vi "ATF-Log command to DR.vi"(8 "error in (no error)":errorcluster, 11 "Cluster":T1) -> (0 "error out":errorcluster)   [LabVIEW 2022 SP3]
uses:
  Controls/SeCrTs-Notifier ctl.ctl
  Controls/SeCrTs-NS Data type.ctl
  Controls/Commands to Log monitor.ctl
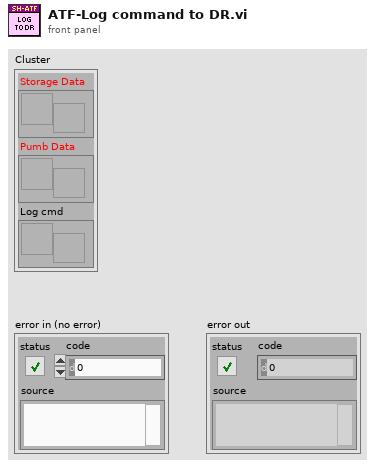
[diagram p1: front panel]
types:
  T1 = typedef "SeCrTs-Notifier ctl.ctl" = cluster{"Storage Data":refnum<notifier>, "Pumb Data":refnum<notifier>, "Log cmd":refnum<notifier>}
  T2 = cluster{"listener ID":refnum<k5>, "connection ID":refnum<k5>, "Log CMD":refnum<notifier>, "Data":cluster{"C/NC":bool, "Start/Stop Log":bool[], "Log Name":string, "Config":cluster{"AO config":cluster{"Channel_Name":string, "Channel_Number":string, "Default_Value":dbl, "Units":string}[], "AI config":cluster{"Channel_Name":string, "Channel_Number":string, "Pre_Scale_min":dbl, "Pre_Scale_max":dbl, "Sensor_min":dbl, "Sensor_max":dbl, "Units":string}[], "DI config":cluster{"Channel_Name":string, "Channel_Number":string, "Default_Value":bool, "DI invert?":bool}[], "DO config":cluster{"Channel_Name":string, "Channel_Number":string, "Default_Value":bool, "DO invert?":bool}[], "TC config":cluster{"Channel_Name":string, "Channel_Number":string, "Pre_Scale_min":dbl, "Pre_Scale_max":dbl, "units":i32, " type":i32}[], "ACC config":cluster{"Channel_Name":string, "Channel_Number":string, "Pre_Scale_min":dbl, "Pre_Scale_max":dbl, "Terminal configuration":i32, "Sensitivity":dbl, "Sensitivity units":i32}[], "SG config":cluster{"Channel_Name":string, "Channel_Number":string, "Pre_Scale_min":dbl, "Pre_Scale_max":dbl}[], "Strain Gauge Settings":cluster{"poisson ratio":dbl, "nominal gage resistance":dbl, "gage factor":dbl}, "Bridge Settings":cluster{"voltage excitation value":dbl, "voltage excitation source":i32, "initial bridge voltage":dbl, "lead wire resistance":dbl, "strain configuration":i32}, "Sample Rate":cluster{"AI Sample Rate":dbl[], "AO Sample Rate":dbl[], "DI Sample Rate":dbl[], "TC Sample Rate":dbl[], "DO Sample Rate":dbl[], "SG Sample Rate":dbl[], "ACC Sample Rate":dbl[]}}, "Log min":dbl}, "timeout":i32}
  T3 = typedef "Commands to Log monitor.ctl" = enum16{"initialize", "Close", "Wait on Listener", "Write", "exit"}
  T4 = cluster{"C/NC":bool, "Start/Stop Log":bool[], "Log Name":string, "Config":cluster{"AO config":cluster{"Channel_Name":string, "Channel_Number":string, "Default_Value":dbl, "Units":string}[], "AI config":cluster{"Channel_Name":string, "Channel_Number":string, "Pre_Scale_min":dbl, "Pre_Scale_max":dbl, "Sensor_min":dbl, "Sensor_max":dbl, "Units":string}[], "DI config":cluster{"Channel_Name":string, "Channel_Number":string, "Default_Value":bool, "DI invert?":bool}[], "DO config":cluster{"Channel_Name":string, "Channel_Number":string, "Default_Value":bool, "DO invert?":bool}[], "TC config":cluster{"Channel_Name":string, "Channel_Number":string, "Pre_Scale_min":dbl, "Pre_Scale_max":dbl, "units":i32, " type":i32}[], "ACC config":cluster{"Channel_Name":string, "Channel_Number":string, "Pre_Scale_min":dbl, "Pre_Scale_max":dbl, "Terminal configuration":i32, "Sensitivity":dbl, "Sensitivity units":i32}[], "SG config":cluster{"Channel_Name":string, "Channel_Number":string, "Pre_Scale_min":dbl, "Pre_Scale_max":dbl}[], "Strain Gauge Settings":cluster{"poisson ratio":dbl, "nominal gage resistance":dbl, "gage factor":dbl}, "Bridge Settings":cluster{"voltage excitation value":dbl, "voltage excitation source":i32, "initial bridge voltage":dbl, "lead wire resistance":dbl, "strain configuration":i32}, "Sample Rate":cluster{"AI Sample Rate":dbl[], "AO Sample Rate":dbl[], "DI Sample Rate":dbl[], "TC Sample Rate":dbl[], "DO Sample Rate":dbl[], "SG Sample Rate":dbl[], "ACC Sample Rate":dbl[]}}, "Log min":dbl}
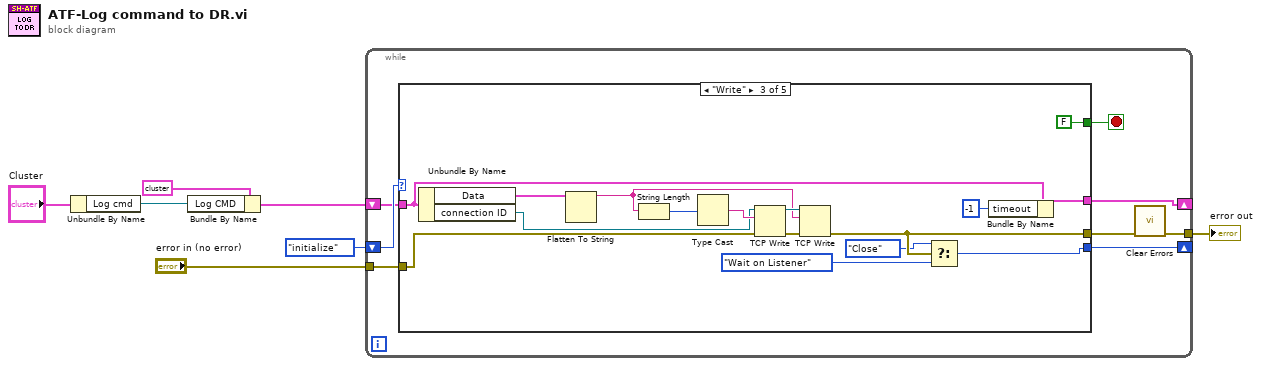
[diagram p0: block diagram]
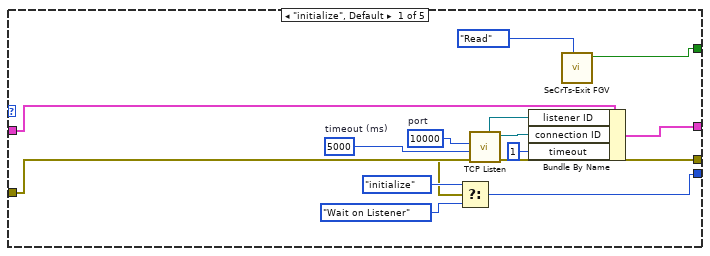
[diagram p2: hidden frame]
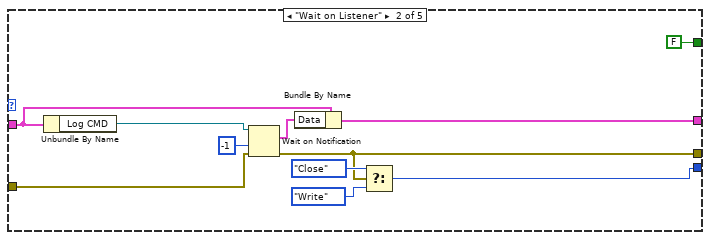
[diagram p3: hidden frame]
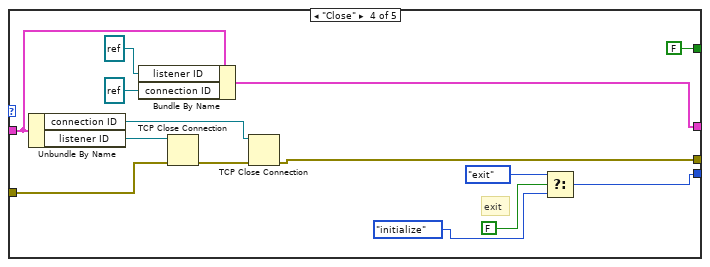
[diagram p4: hidden frame]
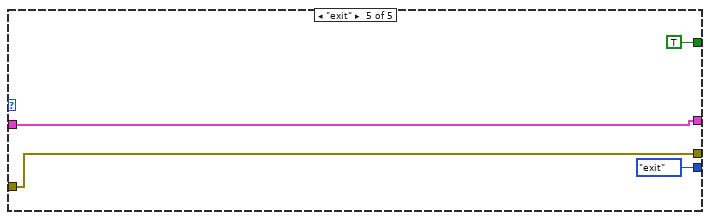
[diagram p5: hidden frame]
diagram:
  n1 = Unbundle By Name("Cluster") -> ("Log cmd"=w1:refnum<notifier>)
  n2 = Bundle By Name(cluster=T2 {"listener ID"=refnum, "connection ID"=refnum, "Log CMD"=refnum, "Data"={"C/NC"=FALSE, "Start/Stop Log"=[], "Log Name"="", "Config"={"AO config"=[], "AI config"=[], "DI config"=[], "DO config"=[], "TC config"=[], "ACC config"=[], "SG config"=[], "Strain Gauge Settings"={"poisson ratio"=0.0, "nominal gage resistance"=0.0, "gage factor"=0.0}, "Bridge Settings"={"voltage excitation value"=0.0, "voltage excitation source"=0, "initial bridge voltage"=0.0, "lead wire resistance"=0.0, "strain configuration"=0}, "Sample Rate"={"AI Sample Rate"=[], "AO Sample Rate"=[], "DI Sample Rate"=[], "TC Sample Rate"=[], "DO Sample Rate"=[], "SG Sample Rate"=[], "ACC Sample Rate"=[]}}, "Log min"=0.0}, "timeout"=-1}, "Log CMD"=w1) -> (w2:T2)
  n3 = while {
    shift-right: [w13] -> _
    shift-left: Commands_to_Log_monitor."initialize" ("Enum") -> [w15]
    tunnel: "error in (no error)" -> [w12]
    tunnel: [w8] -> w5
    shift-right: [w9] -> _
    shift-left: w2 -> [w10]
    stop <- w14 stop-if-true
    n4 = case shown="\"Write\"" w15 {
      tunnel: [w17 FALSE FALSE FALSE TRUE] -> w14
      tunnel: [w26 w32 w47 w60 Commands_to_Log_monitor."exit" ("f")] -> w13
      tunnel: w12 -> [w24 w40 w51 w67 w74]
      tunnel: [w23 w31 w50 w65 w74] -> w11
      tunnel: w10 -> [w21 w37 w42 w63 w71]
      tunnel: [w22 w38 w43 w64 w71] -> w9
      frame "initialize", Default {
        w29 = u16 10000  # port
        w28 = 5000  # timeout (ms)
        n5 = call <vilib>:"TCP Listen.vi"("error in (no error)"=w24, "timeout ms (wait forever: -1)"=w28, "port"=w29) -> ("error out"=w23:errorcluster, "connection ID"=w20:refnum<k5>, "listener ID"=w19:refnum<k5>)  [unwired: 4 in, 2 out]
        n6 = Select(t=Commands_to_Log_monitor."initialize" ("Enum"), s=w23, f=Commands_to_Log_monitor."Wait on Listener") -> (s? t:f=w26:T3)
        n7 = Bundle By Name(cluster=w21, "listener ID"=w19, "connection ID"=w20, "timeout"=1) -> (w22:T2)
        n8 = call "SeCrTs-Exit FGV.vi"("Enum"=enum16{"Init", "Read", "Write"}."Read") -> ("Exit R"=w17:bool)  [unwired: 9 in, 1 out]
      }
      frame "Wait on Listener" {
        n9 = Unbundle By Name(w37) -> ("Log CMD"=w39:refnum<notifier>)
        n10 = Wait on Notification(notifier=w39, timeout in ms (-1)=-1, error in (no error)=w40) -> (notification=w36:T4, error out=w31:errorcluster)  [unwired: 1 in, 2 out]
        n11 = Bundle By Name(cluster=w37, "Data"=w36) -> (w38:T2)
        n12 = Select(t=Commands_to_Log_monitor."Close" ("f"), s=w31, f=Commands_to_Log_monitor."Write") -> (s? t:f=w32:T3)
      }
      frame "Write" {
        n13 = Unbundle By Name(w42) -> ("Data"=w48:T4, "connection ID"=w44:refnum<k5>)
        n14 = Flatten To String(anything=w48) -> (data string=w52:string)  [unwired: 3 in, 2 out]
        n15 = String Length(string=w52) -> (length=w54:i32)
        n16 = Type Cast(x=w54) -> (*(type *) &x=w53:string)  [unwired: 1 out]
        n17 = TCP Write(connection ID=w44, data in=w53, error in (no error)=w51) -> (connection ID out=w56:refnum<k5>, error out=w55:errorcluster)  [unwired: 2 out]
        n18 = TCP Write(connection ID=w56, data in=w52, error in (no error)=w55) -> (error out=w50:errorcluster)  [unwired: 3 out]
        n19 = Select(t=Commands_to_Log_monitor."Close" ("f"), s=w50, f=Commands_to_Log_monitor."Wait on Listener") -> (s? t:f=w47:T3)
        n20 = Bundle By Name(cluster=w42, "timeout"=-1) -> (w43:T2)
      }
      frame "Close" {
        # "exit"
        n21 = Unbundle By Name(w63) -> ("connection ID"=w68:refnum<k5>, "listener ID"=w69:refnum<k5>)
        n22 = Bundle By Name(cluster=w63, "listener ID"=refnum<k5> refnum, "connection ID"=refnum<k5> refnum) -> (w64:T2)
        n23 = TCP Close Connection(connection ID=w69, error in (no error)=w67) -> (error out=w66:errorcluster)  [unwired: 1 in, 1 out]
        n24 = TCP Close Connection(connection ID=w68, error in (no error)=w66) -> (error out=w65:errorcluster)  [unwired: 1 in, 1 out]
        n25 = Select(t=Commands_to_Log_monitor."exit", s=FALSE, f=Commands_to_Log_monitor."initialize") -> (s? t:f=w60:T3)
      }
      frame "exit" {
      }
    }
    n26 = call <vilib>:"Clear Errors.vi"("error in (no error)"=w11) -> ("error out"=w8:errorcluster)  [unwired: 5 in, 1 out]
  }
  "error out" <- w5
